vi "ReadTravelAndForce.vi"(8 "error in":errorcluster, 11 "VISA resource name":refnum<visa-resource-name>) -> (0 "error out":errorcluster, 2 "FeedbackData":T1, 3 "VISA resource name out":refnum<visa-resource-name>)   [LabVIEW 2019, in "Mark 10 TSTM-DC.lvlib"]
uses:
  Mark 10 TSTM-DC.lvlib
  Cluster - FeedbackData.ctl
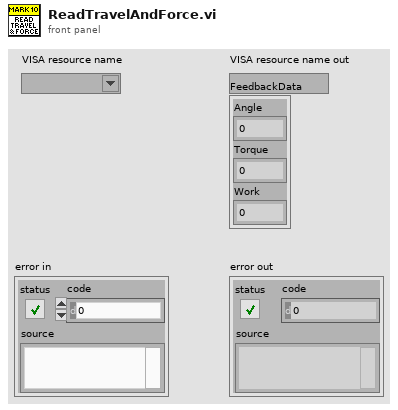
[diagram p1: front panel]
types:
  T1 = typedef "Mark 10 TSTM-DC.lvlib/Cluster - FeedbackData.ctl" = cluster{"Angle":dbl, "Torque":dbl, "Work":dbl}
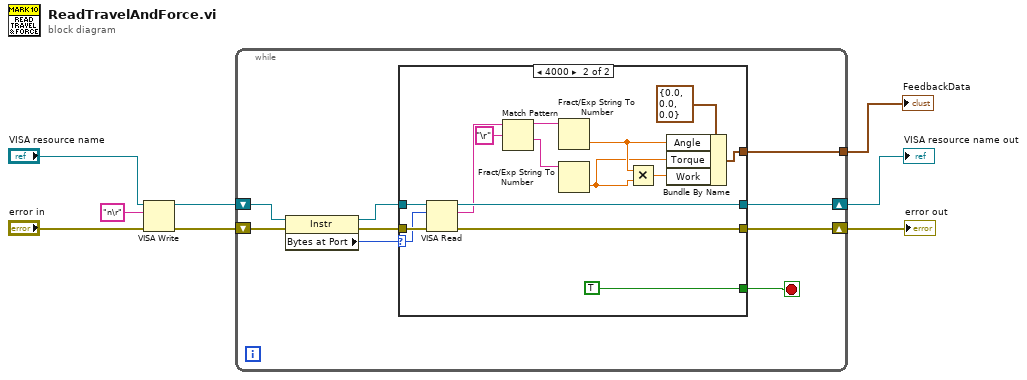
[diagram p0: block diagram]
diagram:
  n1 = VISA Write(VISA resource name="VISA resource name", write buffer="n\r" ("String to Write"), error in (no error)="error in") -> (VISA resource name out=w2:refnum<visa-resource-name>, error out=w3:errorcluster)  [unwired: 1 out]
  n2 = while {
    shift-right: [w13] -> w4
    shift-left: w3 -> [w17]
    shift-right: [w12] -> w7
    shift-left: w2 -> [w15]
    tunnel: [w9] -> w1
    stop <- w10 stop-if-true
    n3 = property class="Instr"(reference=w15, error in=w17) -> (reference out=w14:refnum<visa-resource-name>, error out=w16:errorcluster, "Bytes at Port"=w11:u32)
    n4 = case shown="4000" w11 {
      selector: w11 -> [_ w30]
      tunnel: w16 -> [w18 w34]
      tunnel: w14 -> [w19 w33]
      tunnel: [w18 w32] -> w13
      tunnel: [w19 w31] -> w12
      tunnel: [_ TRUE] -> w10
      tunnel: [_ w23] -> w9
      frame Default {
      }
      frame 4000 {
        n5 = VISA Read(VISA resource name=w33, byte count=w30, error in (no error)=w34) -> (VISA resource name out=w31:refnum<visa-resource-name>, read buffer=w28:string, error out=w32:errorcluster)  [unwired: 1 out]
        n6 = Match Pattern(string=w28, regular expression="\r" ("search string/char (-)")) -> (before substring=w26:string, after substring=w25:string)  [unwired: 1 in, 2 out]
        n7 = Fract/Exp String To Number(string=w26) -> (number=w21:dbl)  [unwired: 3 in, 1 out]
        n8 = Fract/Exp String To Number(string=w25) -> (number=w20:dbl)  [unwired: 3 in, 1 out]
        n9 = Multiply(x=w21, y=w20) -> (x*y=w22:dbl)
        n10 = Bundle By Name(cluster=T1 {"Angle"=0.0, "Torque"=0.0, "Work"=0.0} ("FeedbackData"), "Angle"=w21, "Torque"=w20, "Work"=w22) -> (w23:T1)
      }
    }
  }
  "error out" <- w4
  "VISA resource name out" <- w7
  "FeedbackData" <- w1
